vi "stepper_motor_control_Loop.vi"() -> ()   [LabVIEW 2024]
uses:
  Motor_Type_Def.ctl
  <vilib>/Instr/_visa.llb/Select Event Type.ctl
panel:
  in  "Scan Steps":i32(slide) min=0 max=100 step=1 scale=0.0..100.0
  out "error out":errorcluster
  in  "VISA resource name":refnum<visa-resource-name>="COM5"
  in  "Polarity":bool
  in  "stop":bool
  in  "Move Michelson Motor":bool
  in  "Direction":bool
  in  "Steps":i32(slide)=1 min=1 max=10000 step=1 scale=1.0..10000.0
  in  "Step Time (us)":i32(slide)=100 min=100 max=10000 step=10 scale=100.0..10000.0
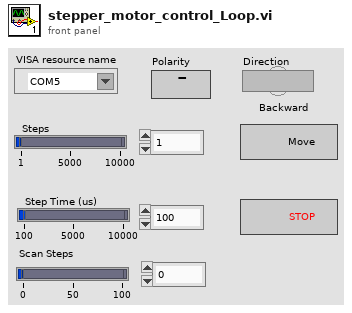
[diagram p1: front panel]
types:
  T1 = typedef "Motor_Type_Def.ctl" = enum16{"Init", "Run"}
  T2 = typedef "Select Event Type.ctl" = u32
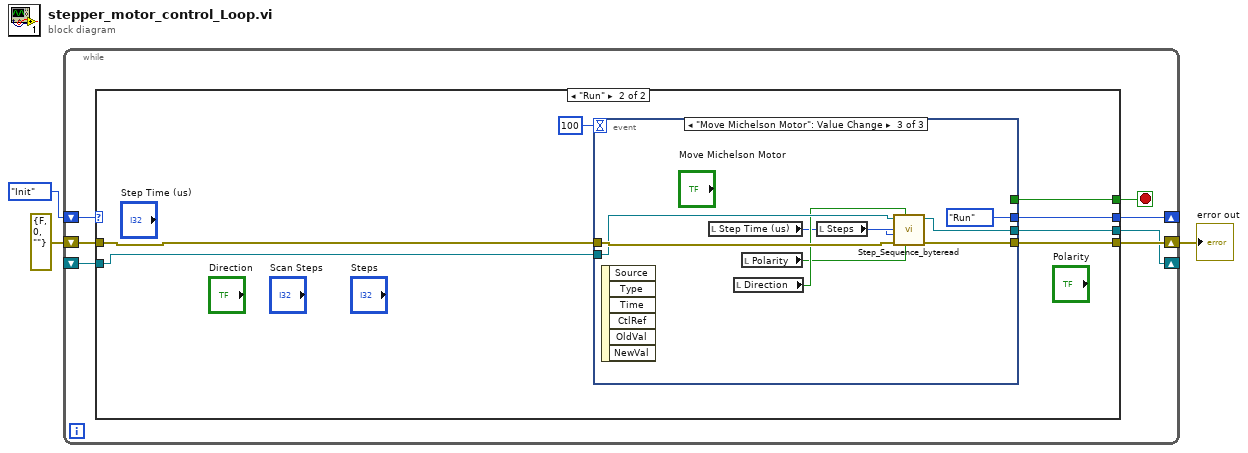
[diagram p0: block diagram]
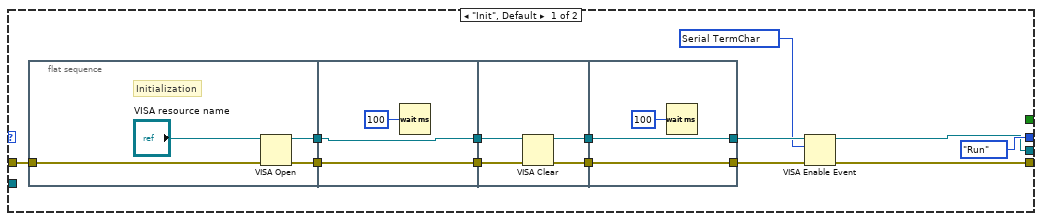
[diagram p2: hidden frame]
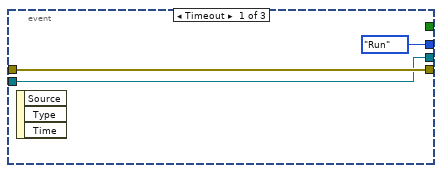
[diagram p3: hidden frame]
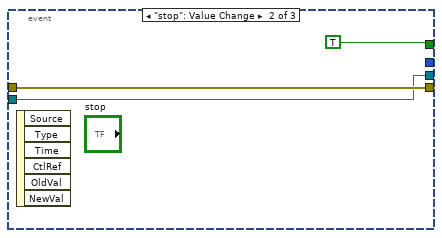
[diagram p4: hidden frame]
diagram:
  n1 = while {
    shift-right: [w9] -> w2
    shift-left: errorcluster {"status"=FALSE, "code"=0, "source"=""} ("error in (no error)") -> [w10]
    shift-right: [w8] -> _
    shift-left: _ -> [w6]
    shift-right: [w5] -> _
    shift-left: Motor_Type_Def."Init" ("Enum") -> [w7]
    stop <- w4 stop-if-true
    n2 = case shown="\"Run\"" w7 {
      tunnel: w10 -> [w17 w44]
      tunnel: [w13 w43] -> w9
      tunnel: [w12 w42] -> w8
      tunnel: w6 -> [_ w39]
      tunnel: [Motor_Type_Def."Run" ("Enum") w40] -> w5
      tunnel: [_ w38] -> w4
      frame "Init", Default {
        w11 = T2 1073684516 items=["Service Request"=1073684491, "Trigger"=3221168138, "Clear"=1073684493, "VXI Signal"=1073684512, "VXI/VME Interrupt"=3221168161, "VXI/VME Sysfail"=1073684509, "VXI/VME Sysreset"=1073684510, "GPIB CIC"=1073684498, "GPIB Talk"=1073684499, "GPIB Listen"=1073684500, "PXI Interrupt"=1073684514, "Serial Break"=1073684515, "Serial TermChar"=1073684516, "Serial CTS"=1073684521, "Serial DSR"=1073684522, "Serial DCD"=1073684524, "Serial RI"=1073684526, "Serial Character"=1073684533, "USB Interrupt"=1073684535, "All Enabled"=1073709055] ("Event Type")
        n3 = flat-sequence {
          tunnel: [w26] -> w23
          tunnel: [w25] -> w22
          tunnel: w17 -> [w24]
          tunnel: [w29] -> w21
          tunnel: w23 -> [w29]
          tunnel: [w28] -> w20
          tunnel: w22 -> [w28]
          tunnel: [w32] -> w19
          tunnel: [w31] -> w18
          tunnel: w21 -> [w34]
          tunnel: w20 -> [w33]
          tunnel: [w36] -> w14
          tunnel: [w37] -> w15
          tunnel: w19 -> [w37]
          tunnel: w18 -> [w36]
          frame #0 {
            # "Initialization"
            n4 = VISA Open(error in (no error)=w24, VISA resource name="VISA resource name") -> (VISA resource name=w25:refnum<visa-resource-name>, error out=w26:errorcluster)  [unwired: 3 in]
          }
          frame #1 {
            n5 = Wait (ms)(milliseconds to wait=u32 100) -> ()  [unwired: 1 out]
          }
          frame #2 {
            n6 = VISA Clear(VISA resource name=w33, error in (no error)=w34) -> (VISA resource name out=w31:refnum<visa-resource-name>, error out=w32:errorcluster)
          }
          frame #3 {
            n7 = Wait (ms)(milliseconds to wait=u32 100) -> ()  [unwired: 1 out]
          }
        }
        n8 = VISA Enable Event(8:w15, 10:w11, 11:w14) -> (0:w13:errorcluster, 3:w12:refnum<visa-resource-name>)  [unwired: 1 in]
      }
      frame "Run" {
        n9 = event shown="[2] \"Move Michelson Motor\": Value Change" {
          selector: _ -> [_ _ _]
          dyn-events: _ -> [_ _ _]
          timeout: 100 -> [_ _ _]
          tunnel: w44 -> [w47 w50 w57]
          tunnel: [w47 w50 w58] -> w43
          tunnel: [w46 w49 w59] -> w42
          tunnel: [Motor_Type_Def."Run" ("Enum") _ Motor_Type_Def."Run" ("Enum")] -> w40
          tunnel: w39 -> [w46 w49 w56]
          tunnel: [_ TRUE _] -> w38
          event Timeout {
            n10 = event-data() -> ()  [unwired: 1 in, 3 out]
          }
          event "stop": Value Change {
            n11 = event-data() -> ()  [unwired: 1 in, 6 out]
          }
          event "Move Michelson Motor": Value Change {
            n12 = event-data() -> ()  [unwired: 1 in, 6 out]
            n13 = local read "Step Time (us)"() -> (w54:i32)
            n14 = local read "Direction"() -> (w55:bool)
            n15 = local read "Polarity"() -> (w51:bool)
            n16 = local read "Steps"() -> (w53:i32)
            n17 = call "Step_Sequence_byteread.vi"("Polarity"=w51, "Direction in"=w55, "error in"=w57, "Steps in"=w53, "Step Time (us) in"=w54, "VISA resource name"=w56) -> ("error out"=w58:errorcluster, "VISA out"=w59:refnum<visa-resource-name>)  [unwired: 4 in]
          }
        }
      }
    }
  }
  "error out" <- w2
